vi "parseDataI32.vi"(8 "error in (no error)":errorcluster, 11 "FrameParser in":refnum<class "DynamicFrameParser.lvclass">) -> (0 "error out":errorcluster, 2 "Data":i32, 3 "FrameParser out":refnum<class "DynamicFrameParser.lvclass">)   [LabVIEW 2016, in "RTModbus.lvlib" / "DynamicFrameParser.lvclass"]
uses:
  DynamicFrameParser.lvclass
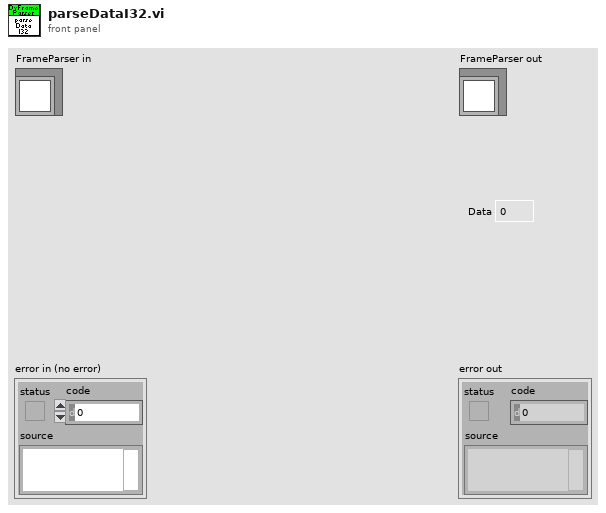
[diagram p1: front panel]
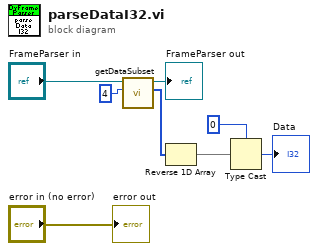
[diagram p0: block diagram]
diagram:
  n1 = call "getDataSubset.vi"("Length"=4 ("Count"), "FrameParser in"="FrameParser in") -> ("Data"=w2:u8[], "FrameParser out"=→"FrameParser out":refnum<class "DynamicFrameParser.lvclass">)  [unwired: 7 in, 1 out]
  n2 = Reverse 1D Array(array=w2) -> (reversed array=w1:u8[])
  n3 = Type Cast(type=0, x=w1) -> (*(type *) &x=→"Data":i32)
  "error out" <- "error in (no error)"
